vi "JSON Tokenizer.vi"(9 "invalid":bool, 10 "string offset":i32, 11 "JSON String":string) -> (2 "Invalid":bool, 3 "Array":T1[](array[typedef]))   [LabVIEW 2020, in "Multi Error Cluster.lvlib"]
doc: "Tokenize the input JSON string just well enough to identify where various JSON tokens are located."
uses:
  <vilib>/MultiError/TokenizeJSON/Multi Error Cluster.lvlib
  <vilib>/MultiError/Errors Cluster Multiple Errors/JSON Token Descriptor.ctl
  <vilib>/MultiError/TokenizeJSON/JSON Raw Token Values.ctl
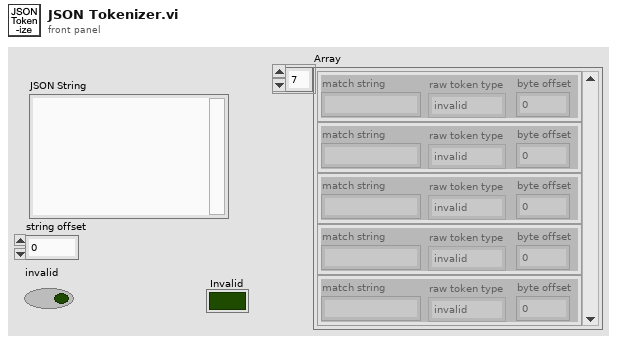
[diagram p1: front panel]
types:
  T1 = typedef "Multi Error Cluster.lvlib/JSON Token Descriptor.ctl" = cluster{"match string":string, "raw token type":T2, "byte offset ":i32}
  T2 = typedef "Multi Error Cluster.lvlib/JSON Raw Token Values.ctl" = enum32{"{", "}", "[", "]", ",", ":", "\"", "number", "string", "true", "false", "null", "invalid"}
  T3 = cluster{"JSON String":string, "token type":T2, "offset past match":i32}
  T4 = cluster{"JSON String":string, "token type":T2, "offset past match":i32}[]
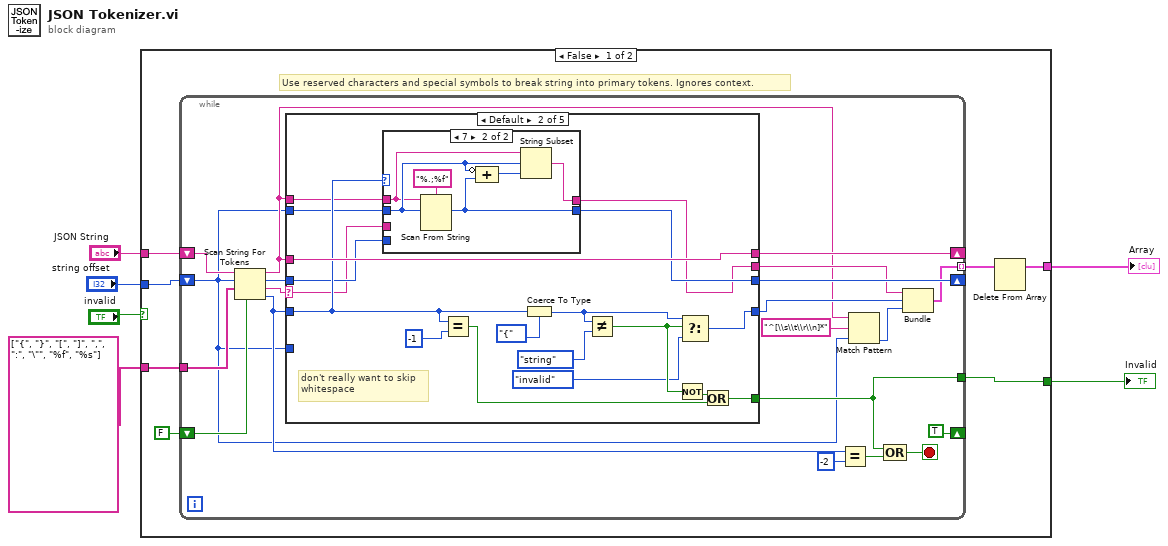
[diagram p0: block diagram]
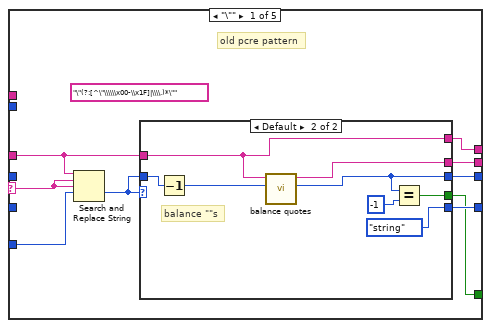
[diagram p2: hidden frame]
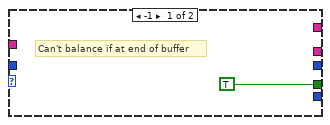
[diagram p3: hidden frame]
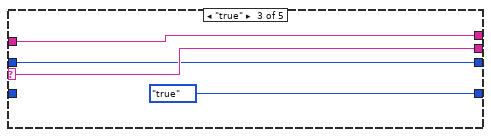
[diagram p5: hidden frame]
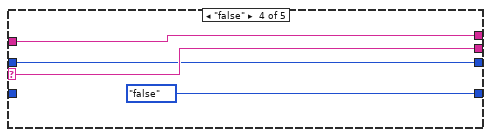
[diagram p6: hidden frame]
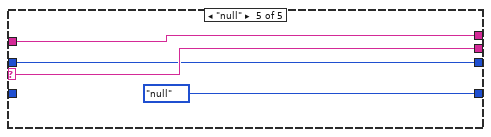
[diagram p7: hidden frame]
diagram:
  n1 = case shown="False" "invalid" {
    selector: "invalid" -> [_ w90]
    tunnel: "string offset" -> [w12 _]
    tunnel: "JSON String" -> [w11 _]
    tunnel: [w9 _] -> w4
    tunnel: [w7 w90] -> w3
    tunnel: string[] ["{", "}", "[", "]", ",", ":", "\"", "%f", "%s"] ("operators (none)") -> [w8 _]
    frame False {
      # "Use reserved characters and special symbols to break string into primary tokens. Ignores context."
      n2 = while {
        shift-right: [w27] -> _
        shift-left: w11 -> [w33]
        shift-right: [w26] -> _
        shift-left: w12 -> [w14]
        shift-right: [TRUE] -> _
        shift-left: FALSE -> [w32]
        tunnel: [w22] -> w10 mode=indexing
        tunnel: [w17] -> w7
        tunnel: w8 -> [w16]
        stop <- w18 stop-if-true
        n3 = Scan String For Tokens(4:w32, 7:w16, 8:w14, 9:w33) -> (0:w25:i32, 1:w29:string, 2:w28:i32, 3:w15:string)  [unwired: 2 in]
        n4 = case shown="Default" w29 {
          selector: w29 -> [w34 w55 w81 w85 w89]
          tunnel: w15 -> [w37 w59 w80 w84 w88]
          tunnel: w28 -> [_ w56 w79 w83 w87]
          tunnel: [w38 w59 w80 w84 w88] -> w27
          tunnel: [w40 w57 w79 w83 w87] -> w26
          tunnel: [w42 w54 w81 w85 w89] -> w24
          tunnel: w25 -> [_ w58 _ _ _]
          tunnel: [w41 w68 JSON_Raw_Token_Values."true" ("token type") JSON_Raw_Token_Values."false" ("token type") JSON_Raw_Token_Values."null" ("token type")] -> w23
          tunnel: [w39 w62 _ _ _] -> w17
          tunnel: w14 -> [w36 _ _ _ _]
          tunnel: w15 -> [_ w53 _ _ _]
          tunnel: w14 -> [_ w52 _ _ _]
          frame "\"" {
            (unwired) "\"(?:[^\"\\\\\\x00-\\x1F]|\\\\.)*\"" ("regular expression")
            # "old pcre pattern"
            n5 = Search and Replace String(input string=w37, search string=w34, replace string=w34, offset=w36) -> (offset past replacement=w35:i32)  [unwired: 4 in, 3 out]
            n6 = case shown="Default" w35 {
              tunnel: w35 -> [_ w51]
              tunnel: [_ w44] -> w42
              tunnel: w37 -> [_ w47]
              tunnel: [_ JSON_Raw_Token_Values."string" ("token type")] -> w41
              tunnel: [_ w45] -> w40
              tunnel: [TRUE w49] -> w39
              tunnel: [_ w47] -> w38
              frame -1 {
                # "Can't balance if at end of buffer"
              }
              frame Default {
                # "balance \"\"s"
                n7 = Decrement(x=w51) -> (x-1=w46:i32)
                n8 = call <vilib>:"balance quotes.vi"("offset"=w46, "string"=w47) -> ("offset out"=w45:i32, "quoted string"=w44:string)  [unwired: 8 in]
                n9 = Equal?(x=w45, y=-1) -> (x = y?=w49:bool)
              }
            }
          }
          frame Default {
            # "don't really want to skip\nwhitespace"
            n10 = case shown="7" w58 {
              tunnel: w55 -> [w70 _]
              tunnel: [w71 w75] -> w57
              tunnel: w56 -> [w71 _]
              tunnel: [w70 w76] -> w54
              tunnel: w53 -> [_ w72]
              tunnel: w52 -> [_ w74]
              frame Default {
              }
              frame 7 {
                n11 = Scan From String(format string="%.;%f", input string=w72, initial scan location=w74) -> (offset past scan=w75:u32)  [unwired: 3 in, 2 out]
                n12 = Compound Arithmetic op=ADD(invert w74, w75) -> (w73:u32)
                n13 = String Subset(string=w72, offset (0)=w74, length (rest)=w73) -> (substring=w76:string)
              }
            }
            n14 = Equal?(x=w58, y=-1) -> (x = y?=w60:bool)
            n15 = Coerce To Type(0:w58, 1:JSON_Raw_Token_Values."{" ("token type")) -> (2:w69:T2)
            n16 = Not Equal?(x=w69, y=JSON_Raw_Token_Values."string" ("token type")) -> (x != y?=w67:bool)
            n17 = Not(x=w67) -> (.not. x?=w61:bool)
            n18 = Select(t=w69, s=w67, f=JSON_Raw_Token_Values."invalid" ("token type")) -> (s? t:f=w68:T2)
            n19 = Or(x=w61, y=w60) -> (x .or. y?=w62:bool)
          }
          frame "true" {
          }
          frame "false" {
          }
          frame "null" {
          }
        }
        n20 = Equal?(x=w25, y=-2) -> (x = y?=w19:bool)
        n21 = Match Pattern(string=w15, regular expression="^[\\s\\t\\r\\n]*", offset (0)=w14) -> (offset past match=w20:i32)  [unwired: 3 out]
        n22 = Compound Arithmetic op=OR(w17, w19) -> (w18:bool)
        n23 = Bundle("JSON String"=w24, "token type"=w23, "offset past match"=w20) -> (w22:T3)  [unwired: 1 in]
      }
      n24 = Delete From Array(array=w10) -> (array with subset deleted=w9:T4)  [unwired: 2 in, 1 out]
    }
    frame True {
    }
  }
  "Invalid" <- w3
  "Array" <- w4
